vi "SearchTimestampArray.vi"(8 "Timestamp Array":u32[](array[numeric]), 11 "Search Timestamp":u32) -> (0 "Index of Minimum":i32, 3 "Index of Maximum":i32)   [LabVIEW 2020]
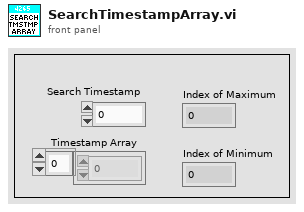
[diagram p1: front panel]
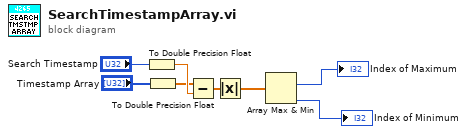
[diagram p0: block diagram]
diagram:
  n1 = To Double Precision Float(number="Search Timestamp") -> (double precision float=w8:dbl)
  n2 = To Double Precision Float(number="Timestamp Array") -> (double precision float=w3:dbl[])
  n3 = Subtract(x=w3, y=w8) -> (x-y=w4:dbl[])
  n4 = Absolute Value(x=w4) -> (abs(x)=w5:dbl[])
  n5 = Array Max & Min(array=w5) -> (max index (indices)=→"Index of Maximum":i32, min index (indices)=→"Index of Minimum":i32)  [unwired: 2 out]
